vi "GetDI.vi"(3 "error in (no error)":errorcluster, 5 "VISA resource":refnum<visa-resource-name>="COM1") -> (0 "error out":errorcluster, 1 "DI(=CTS) State":i16 min=0 max=1 step=1, 2 "dup VISA resource":refnum<visa-resource-name>="COM1")   [LabVIEW 2021]
doc: "Reads state of data signal\nfrom AVS-47B"
panel:
  # "GetDI.vi"
  # "This VI reads  the state (1 or 0)  of the DI  (Data from Instrument)  Picobus input  line  (CTS  handshake of COM port)."
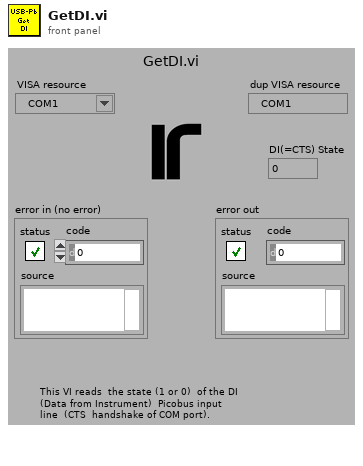
[diagram p1: front panel]
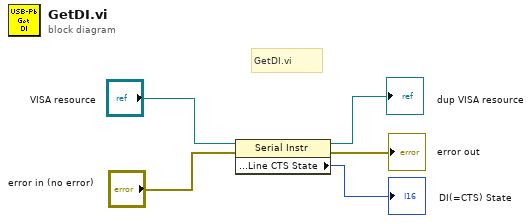
[diagram p0: block diagram]
diagram:
  # "GetDI.vi"
  n1 = property class="Serial Instr"(reference="VISA resource", error in="error in (no error)") -> (reference out=→"dup VISA resource":refnum<visa-resource-name>, error out=→"error out":errorcluster, "Serial Settings:Modem Line Settings:Line CTS State"=→"DI(=CTS) State":i16)
